vi "Handle Error.vi"(7 "Stop on Unhandled Error (T)":bool=TRUE, 8 "error in":errorcluster, 11 "Instrument.Oxford1820":refnum<class "Instrument.Oxford1820.lvclass">) -> (0 "handling error":errorcluster, 2 "Unhandled error":errorcluster, 3 "Instrument.Oxford1820 out":refnum<class "Instrument.Oxford1820.lvclass">)   [LabVIEW 2019, in "Instrument.Oxford1820.lvclass"]
doc: "JKI State Machine Objects (SMO) 1.0.0.11\nJKI - JKI\nCopyright (c) 2016, JKI"
uses:
  Instrument.Oxford1820.lvclass
  Instrument.Oxford1820.lvclass/Instrument.Oxford1820.ctl
  <userlib>/LevyLab/Instrument Framework/Instrument Types/Cryostat/Instrument.Cryostat.lvclass
panel:
  # "For instructions on how to use the JKI State Machine Objects, examples and video tutorials, visit:\nhttp://jki.net/state-machine-objects/\n\nJKI State Machine Objects™\nhttp://jki.net/state-machine-objects/\nCopyright (C) 2005-2015, JKI <info@jki.net>\nALL RIGHTS RESERVED"
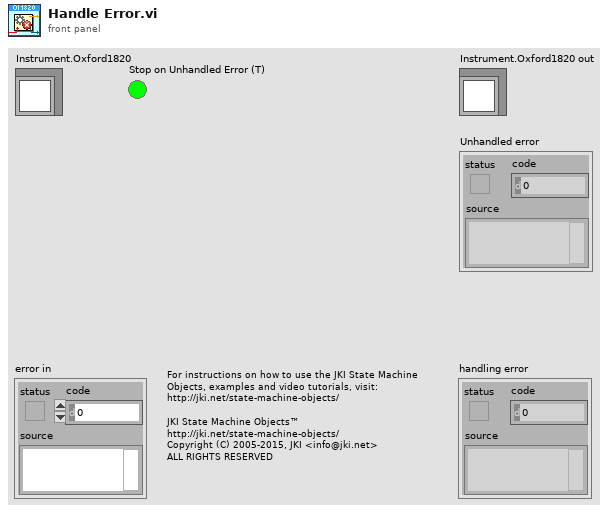
[diagram p1: front panel]
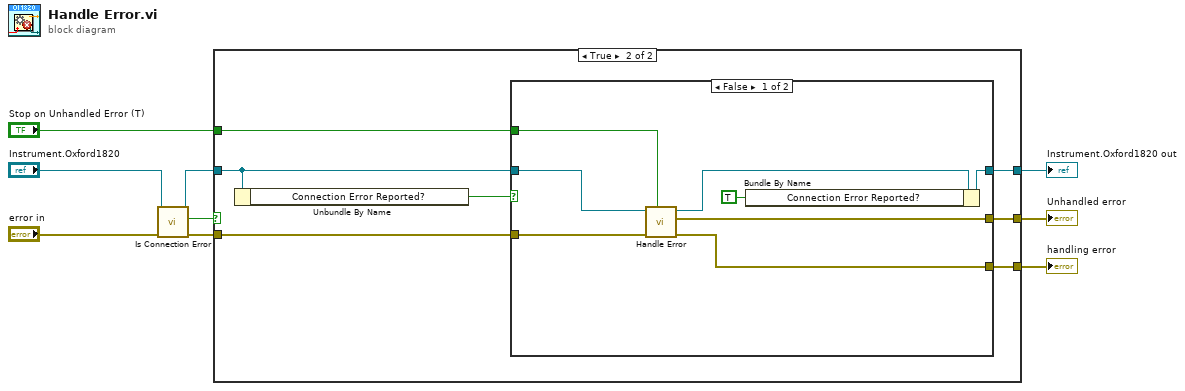
[diagram p0: block diagram]
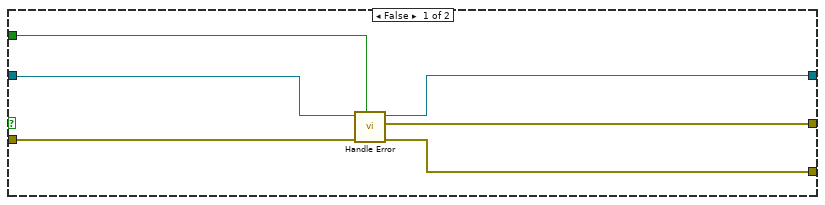
[diagram p2: hidden frame]
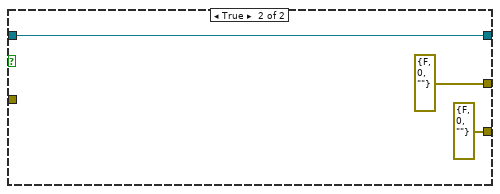
[diagram p3: hidden frame]
diagram:
  n1 = call "Is Connection Error.vi"("error in (no error)"="error in", "Instrument.Oxford1820 in"="Instrument.Oxford1820") -> ("error out"=w2:errorcluster, "Connection Error?"=w1:bool, "Instrument.Oxford1820 out"=w3:refnum<class "Instrument.Oxford1820.lvclass">)  [unwired: 7 in]
  n2 = case shown="True" w1 {
    tunnel: [w10 w22] -> w9
    tunnel: [w11 w21] -> w8
    tunnel: [w12 w20] -> w7
    tunnel: "Stop on Unhandled Error (T)" -> [w13 w19]
    tunnel: w3 -> [w14 w17]
    tunnel: w2 -> [w15 w16]
    frame False {
      n3 = call-parent "Handle Error.vi"("Stop on Unhandled Error (T)"=w13, "error in"=w15, "SMO"=w14) -> ("handling error"=w10:errorcluster, "Unhandled error"=w11:errorcluster, "SMO out"=w12:refnum<class "Instrument.Oxford1820.lvclass">)  [unwired: 6 in]
    }
    frame True {
      n4 = Unbundle By Name(w17) -> ("Connection Error Reported?"=w18:bool)
      n5 = case shown="False" w18 {
        tunnel: [w30 errorcluster {"status"=FALSE, "code"=0, "source"=""} ("handling error")] -> w22
        tunnel: [w29 errorcluster {"status"=FALSE, "code"=0, "source"=""} ("Unhandled error")] -> w21
        tunnel: [w25 w33] -> w20
        tunnel: w19 -> [w28 _]
        tunnel: w16 -> [w27 _]
        tunnel: w17 -> [w26 w33]
        frame False {
          n6 = call-parent "Handle Error.vi"("Stop on Unhandled Error (T)"=w28, "error in"=w27, "SMO"=w26) -> ("handling error"=w30:errorcluster, "Unhandled error"=w29:errorcluster, "SMO out"=w23:refnum<class "Instrument.Oxford1820.lvclass">)  [unwired: 6 in]
          n7 = Bundle By Name(cluster=w23, "Connection Error Reported?"=TRUE ("Connection.Connection Error Reported?")) -> (w25:refnum<class "Instrument.Oxford1820.lvclass">)
        }
        frame True {
        }
      }
    }
  }
  "handling error" <- w9
  "Instrument.Oxford1820 out" <- w7
  "Unhandled error" <- w8
